vi "Init.vi"(8 "error in (no error)":errorcluster, 11 "Santec in":refnum<class "Santec.lvclass">) -> (0 "error out":errorcluster, 3 "Santec out":refnum<class "Santec.lvclass">)   [LabVIEW 2015, in "Santec.lvclass"]
uses:
  Santec.lvclass
  Laser.lvclass
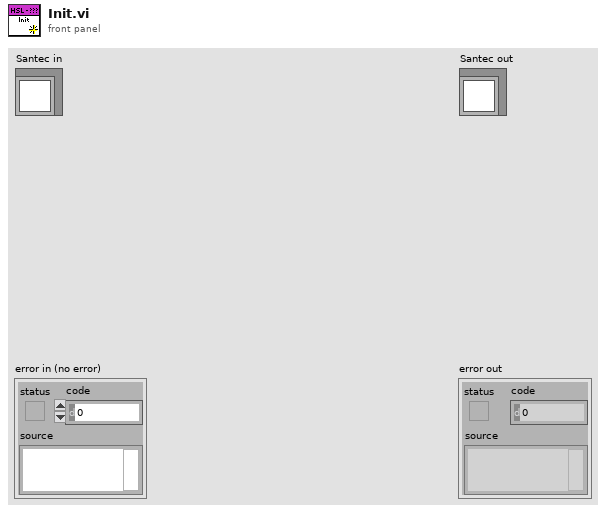
[diagram p1: front panel]
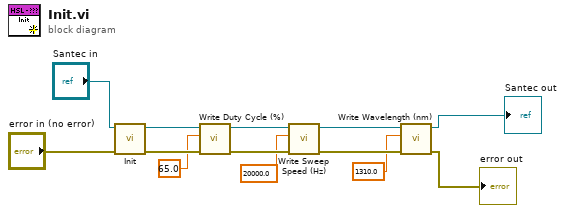
[diagram p0: block diagram]
diagram:
  n1 = call-parent "Init.vi"("error in (no error)"="error in (no error)", "Laser in"="Santec in") -> ("error out"=w11:errorcluster, "Laser out"=w10:refnum<class "Santec.lvclass">)  [unwired: 8 in]
  n2 = call-dynamic "Write Duty Cycle (%).vi"("error in (no error)"=w11, "Duty Cycle (%)"=65.0, "Laser in"=w10) -> ("error out"=w8:errorcluster, "Laser out"=w9:refnum<class "Santec.lvclass">)  [unwired: 7 in]
  n3 = call-dynamic "Write Sweep Speed (Hz).vi"("error in (no error)"=w8, "Sweep Speed (Hz)"=20000.0, "Laser in"=w9) -> ("error out"=w7:errorcluster, "Laser out"=w6:refnum<class "Santec.lvclass">)  [unwired: 7 in]
  n4 = call-dynamic "Write Wavelength (nm).vi"("error in (no error)"=w7, "Wavelength (nm)"=1310.0, "Laser in"=w6) -> ("error out"=→"error out":errorcluster, "Laser out"=→"Santec out":refnum<class "Santec.lvclass">)  [unwired: 7 in]
